vi "Execute Start Real.vi"(4 "Menu Item Tag Suffix":string, 6 "相对位置原点":T1 caption="位置", 7 "Insert?":bool, 8 "错误输入（无错误）":errorcluster, 10 "所有者引用句柄":refnum<vi>, 11 "接线端输入":refnum<vi>) -> (0 "错误输出":errorcluster)   [LabVIEW 2020]
uses:
  <vilib>/Utility/miscctls.llb/LVPointTypeDef.ctl
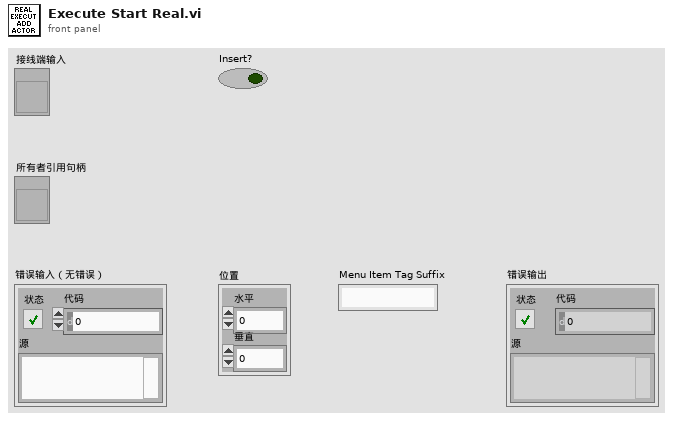
[diagram p1: front panel]
types:
  T1 = typedef "LVPointTypeDef.ctl" = cluster{"Horizontal":i16, "Vertical":i16}
  T2 = typedef "LVRectTypeDef.ctl" = cluster{"Left":i16, "Top":i16, "Right":i16, "Bottom":i16}
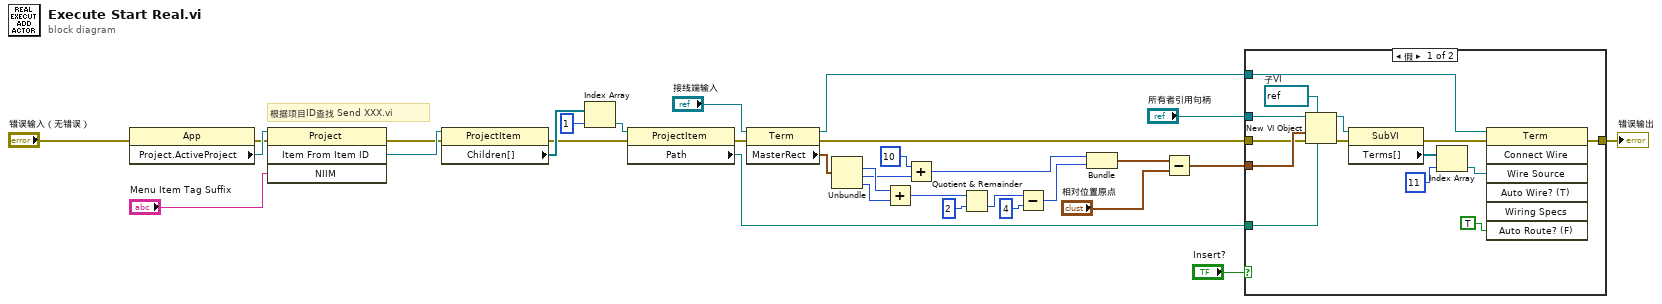
[diagram p0: block diagram]
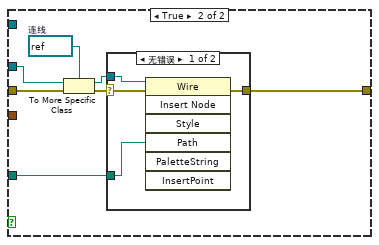
[diagram p2: hidden frame]
diagram:
  # "根据项目ID查找 Send XXX.vi"
  n1 = property class="App"(error in="错误输入（无错误）") -> (error out=w24:errorcluster, "Project.ActiveProject"=w29:refnum<vi>)  [unwired: 1 in, 1 out]
  n2 = invoke class="Project" method="Item From Item ID"(reference=w29, error in=w24, "NIIM"="Menu Item Tag Suffix") -> (error out=w23:errorcluster, "GetItemFromNIIM"=w28:refnum<vi>)  [unwired: 1 in, 2 out]
  n3 = property class="ProjectItem"(reference=w28, error in=w23) -> (error out=w22:errorcluster, "Children[]"=w26:refnum<vi>[])  [unwired: 1 out]
  n4 = Index Array(array=w26, index=1) -> (element=w27:refnum<vi>)
  n5 = property class="ProjectItem"(reference=w27, error in=w22) -> (error out=w21:errorcluster, "Path"=w32:path)  [unwired: 1 out]
  n6 = property class="Term"(reference="接线端输入", error in=w21) -> (reference out=w15:refnum<vi>, error out=w17:errorcluster, "MasterRect"=w6:T2)
  n7 = Unbundle(w6) -> ("Top"=w13:i16, "Right"=w2:i16, "Bottom"=w12:i16)  [unwired: 1 out]
  n8 = Add(x=w13, y=w12) -> (x+y=w11:i16)
  n9 = Add(x=i16 10 ("y"), y=w2) -> (x+y=w14:i16)
  n10 = Quotient & Remainder(x=w11, y=i16 2) -> (floor(x/y)=w8:i16)  [unwired: 1 out]
  n11 = Subtract(x=w8, y=i16 4) -> (x-y=w7:i16)
  n12 = Bundle(w14, w7) -> (w5:cluster{i16, i16})  [unwired: 1 in]
  n13 = Subtract(x=w5, y="相对位置原点") -> (x-y=w3:T1)
  n14 = case shown="假" "Insert?" {
    tunnel: w32 -> [w46 w48]
    tunnel: w15 -> [w45 _]
    tunnel: "所有者引用句柄" -> [w44 w50]
    tunnel: w3 -> [w37 _]
    tunnel: w17 -> [w36 w52]
    tunnel: [w33 w47] -> w20
    frame False {
      w43 = refnum<vi> refnum  # 子VI
      n15 = New VI Object(vi object class=w43, owner refnum=w44, position/next to=w37, 6:w46, 8:w36) -> (object refnum=w39:refnum<vi>, 0:w35:errorcluster)  [unwired: 3 in]
      n16 = property class="SubVI"(reference=w39, error in=w35) -> (error out=w34:errorcluster, "Terms[]"=w38:refnum<vi>[])  [unwired: 1 out]
      n17 = Index Array(array=w38, index=11) -> (element=w40:refnum<vi>)
      n18 = invoke class="Term" method="Connect Wire"(reference=w45, error in=w34, "Wire Source"=w40, "Auto Route? (F)"=TRUE ("自动查找路径？(F)")) -> (error out=w33:errorcluster)  [unwired: 3 in, 6 out]
    }
    frame True {
      w53 = refnum<vi> refnum  # 连线
      n19 = To More Specific Class(target class=w53, reference=w50, error in=w52) -> (specific class reference=w49:refnum<vi>, error out=w51:errorcluster)
      n20 = case shown="无错误" w51 {
        selector: w51 -> [w57 w58]
        tunnel: w49 -> [w56 _]
        tunnel: w48 -> [w55 _]
        tunnel: [w54 w58] -> w47
        frame No Error {
          n21 = invoke class="Wire" method="Insert Node"(reference=w56, error in=w57, "Path"=w55) -> (error out=w54:errorcluster)  [unwired: 4 in, 6 out]
        }
        frame Error {
        }
      }
    }
  }
  "错误输出" <- w20
